vi "WAIT.vi"(10 "argv":string[](array[string]), 11 "args":u8) -> ()   [LabVIEW 2011]
uses:
  <vilib>/Rock Robotics/WPI/DriverStation/WPI_DriverStationStatusErrorCache.ctl
  Auto_Conf.vi
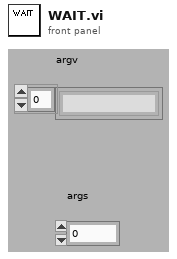
[diagram p1: front panel]
types:
  T1 = typedef "WPI_DriverStationStatusErrorCache.ctl" = enum16{"Get", "Set"}
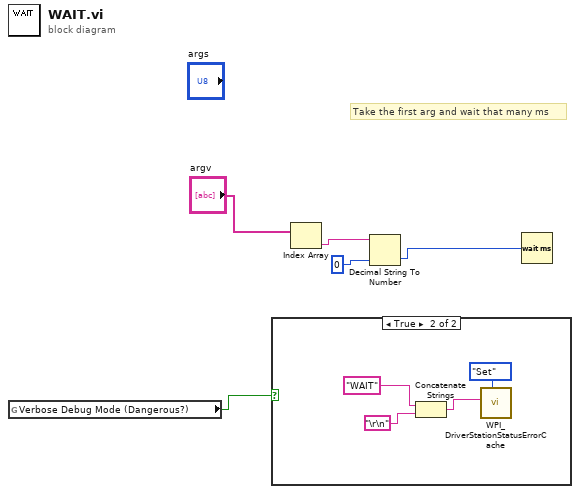
[diagram p0: block diagram]
diagram:
  # "Take the first arg and wait that many ms"
  n1 = global read "Auto_Conf.vi" "Verbose Debug Mode (Dangerous?)"() -> (w1:bool)
  n2 = case shown="True" w1 {
    frame False {
    }
    frame True {
      n3 = Concatenate Strings("WAIT" ("string"), "\r\n") -> (w7:string)
      n4 = call <vilib>:"WPI_DriverStationStatusErrorCache.vi"("StatusErrorCacheOp"=WPI_DriverStationStatusErrorCache."Set", "Error String"=w7) -> ()  [unwired: 10 out]
    }
  }
  n5 = Index Array(array="argv") -> (element=w4:string)  [unwired: 1 in]
  n6 = Decimal String To Number(string=w4, default (0L)=u32 0 ("milliseconds to wait")) -> (number=w2:u32)  [unwired: 2 out]
  n7 = Wait (ms)(milliseconds to wait=w2) -> ()  [unwired: 1 out]
